vi "Memory.Pointer.Read Bytes.In Place.Safe.vi"(8 "error in (no error)":errorcluster, 10 "buffer in":u8[](array[numeric]) format="%02x", 11 "Pointer in":refnum<class "Memory.Pointer.Void.lvclass">) -> (0 "error out":errorcluster, 2 "buffer out":u8[](array[numeric]) format="%02x", 3 "Pointer out":refnum<class "Memory.Pointer.Void.lvclass">)   [LabVIEW 2016, in "Memory Manager.lvlib" / "Memory.Pointer.Void.lvclass"]
uses:
  Memory.Pointer.Void.lvclass
  Memory.Pointer.Void.lvclass/Memory.Pointer.Void.ctl
  Memory.Pointer.Get Address.vi
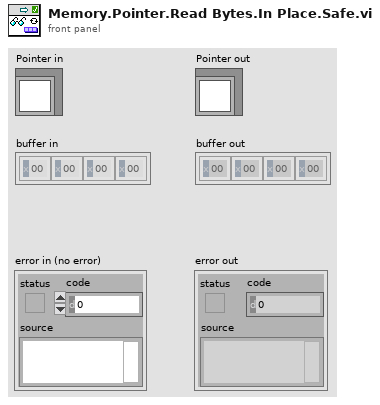
[diagram p1: front panel]
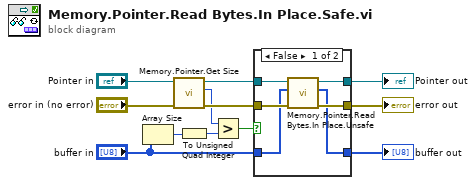
[diagram p0: block diagram]
diagram:
  n1 = Array Size(array="buffer in") -> (size(s)=w7:i32)
  n2 = call "Memory.Pointer.Get Size.vi"("error in (no error)"="error in (no error)", "Pointer in"="Pointer in") -> ("error out"=w3:errorcluster, "size"=w1:u64, "Pointer out"=w5:refnum<class "Memory.Pointer.Void.lvclass">)  [unwired: 7 in]
  n3 = To Unsigned Quad Integer(1:w7) -> (0:w6:u64)
  n4 = Greater?(x=w1, y=w6) -> (0:w8:bool)
  n5 = case shown="False" w8 {
    tunnel: [w13 w21] -> w12
    tunnel: "buffer in" -> [w14 w21]
    tunnel: w5 -> [w18 w20]
    tunnel: [w16 w20] -> w4
    tunnel: w3 -> [w17 w19]
    tunnel: [w15 w19] -> w2
    frame False {
      n6 = call "Memory.Pointer.Read Bytes.In Place.Unsafe.vi"("error in (no error)"=w17, "buffer in"=w14, "Pointer in"=w18) -> ("error out"=w15:errorcluster, "buffer out"=w13:u8[], "Pointer out"=w16:refnum<class "Memory.Pointer.Void.lvclass">)  [unwired: 6 in]
    }
    frame True {
      # "#TODO\nThrow error."
    }
  }
  "error out" <- w2
  "Pointer out" <- w4
  "buffer out" <- w12
